vi "Get_DevicesInformation.vi"(8 "error in (no error)":errorcluster, 11 "Abstract_Mono in":refnum<class "Abstract_Mono.lvclass">) -> (0 "error out":errorcluster, 2 "Array":string[](array[string]), 3 "Abstract_Mono out":refnum<class "Abstract_Mono.lvclass">)   [LabVIEW 2020, in "Abstract_Mono.lvclass"]
uses:
  <instrlib>/Classes/Monochromator/Monochromator_Abstract/Abstract_Mono.lvclass
panel:
  in  "Ring":u16(ring) items=["Front"=0, "Side"=1, "Not Defined"=100]
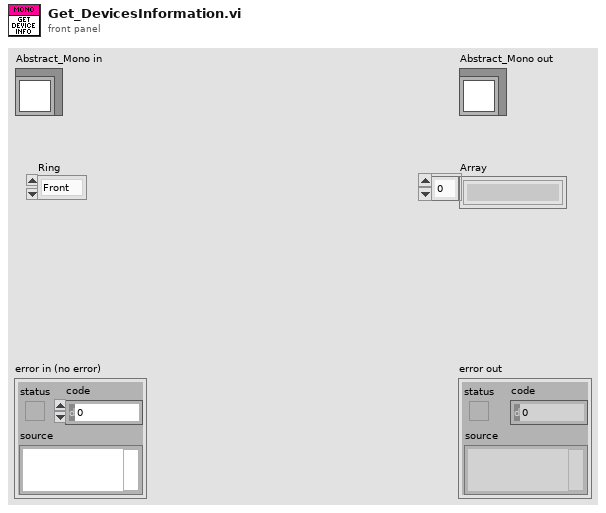
[diagram p1: front panel]
types:
  T1 = typedef "LVStringsAndValuesArrayTypeDef_U16.ctl" = cluster{"String":string, "Value":u16}[]
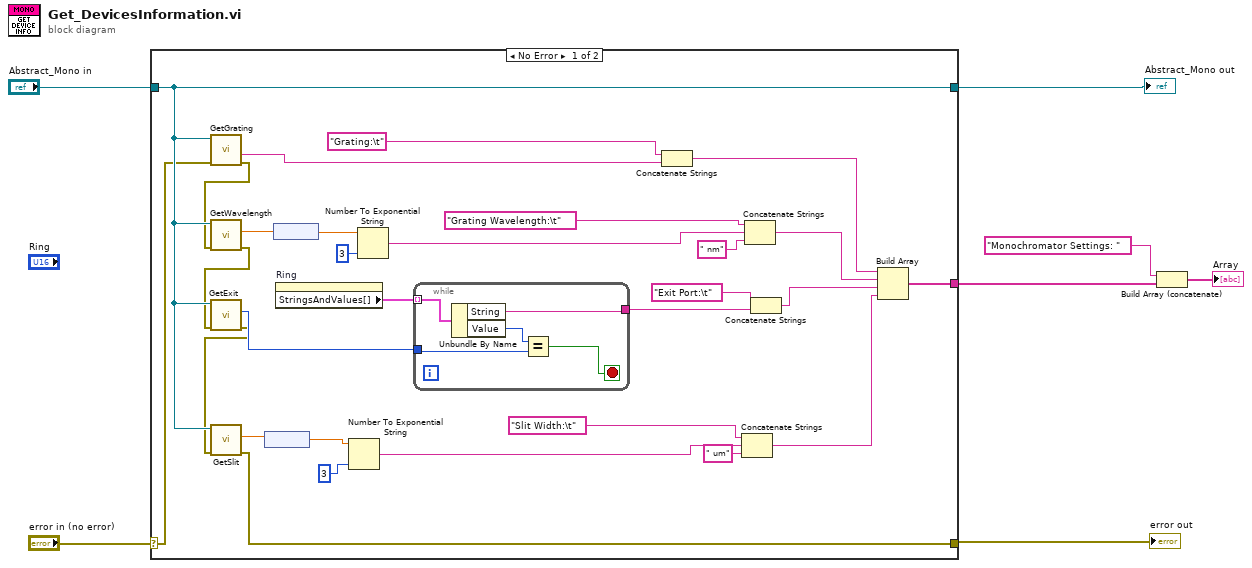
[diagram p0: block diagram]
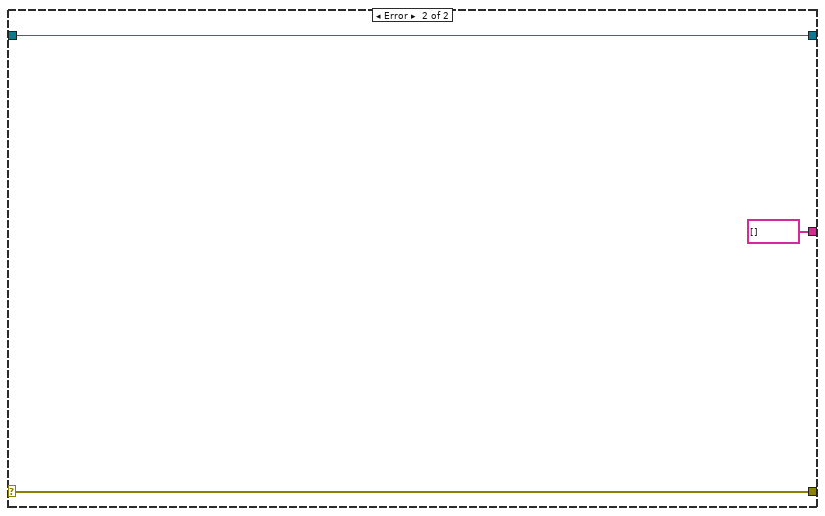
[diagram p2: hidden frame]
diagram:
  n1 = case shown="No Error" "error in (no error)" {
    selector: "error in (no error)" -> [w12 w44]
    tunnel: [w8 w44] -> w6
    tunnel: [w36 w43] -> w4
    tunnel: "Abstract_Mono in" -> [w36 w43]
    tunnel: [w13 string[] []] -> w2
    frame No Error {
      n2 = call-dynamic "GetGrating.vi"("error in (no error)"=w12, "Abstract_Mono in"=w36) -> ("error out"=w11:errorcluster, "Grating Name"=w26:string)  [unwired: 6 in, 2 out]
      n3 = call-dynamic "GetWavelength.vi"("error in (no error)"=w11, "Abstract_Mono in"=w36) -> ("error out"=w10:errorcluster, "Numeric"=w35:dbl[unit])  [unwired: 7 in, 1 out]
      n4 = call-dynamic "GetExit.vi"("error in (no error)"=w10, "Abstract_Mono in"=w36) -> ("error out"=w9:errorcluster, "Ring"=w31:u16)  [unwired: 7 in, 1 out]
      n5 = call-dynamic "GetSlit.vi"("error in (no error)"=w9, "Abstract_Mono in"=w36) -> ("error out"=w8:errorcluster, "Numeric"=w30:dbl[unit])  [unwired: 7 in, 1 out]
      n6 = node(w30) -> (w28:dbl)
      n7 = node(w35) -> (w34:dbl)
      n8 = property on="Ring" class="Ring (strict)"() -> ("StringsAndValues[]"=w32:T1)  [unwired: 2 in, 2 out]
      n9 = Number To Exponential String(number=w28, precision (6)=i16 3) -> (E-format string=w19:string)  [unwired: 2 in]
      n10 = Number To Exponential String(number=w34, precision (6)=i16 3) -> (E-format string=w24:string)  [unwired: 2 in]
      n11 = while {
        tunnel: w32 -> [w41] mode=indexing
        tunnel: w31 -> [w39]
        tunnel: [w37] -> w21
        stop <- w38 stop-if-true
        n12 = Unbundle By Name(w41) -> ("String"=w37:string, "Value"=w40:u16)
        n13 = Equal?(x=w40, y=w39) -> (x = y?=w38:bool)
      }
      n14 = Concatenate Strings("Grating:\t", w26) -> (w17:string)
      n15 = Concatenate Strings("Slit Width:\t", w19, " um" ("string")) -> (w14:string)
      n16 = Concatenate Strings("Grating Wavelength:\t", w24, " nm" ("string")) -> (w16:string)
      n17 = Concatenate Strings("Exit Port:\t", w21) -> (w15:string)
      n18 = Build Array(w17, w16, w15, w14) -> (w13:string[])
    }
    frame Error {
    }
  }
  "error out" <- w6
  "Abstract_Mono out" <- w4
  n19 = Build Array (concatenate)("Monochromator Settings: ", w2) -> (→"Array":string[])
